vi "getSubM.vi"(9 "Index of Raws":T1, 11 "3D Array":dbl[][][](array[numeric])) -> (3 "Sub-Array":dbl[][][](array[numeric]))   [LabVIEW 2016]
doc: "Get the sub-matrix from a 3D matrix."
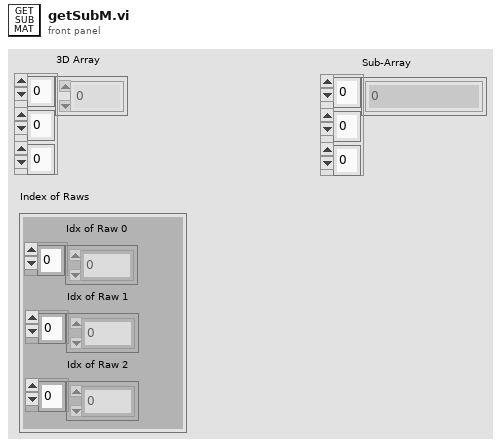
[diagram p1: front panel]
types:
  T1 = cluster{"Idx of Raw 0":i32[], "Idx of Raw 1":i32[], "Idx of Raw 2":i32[]}
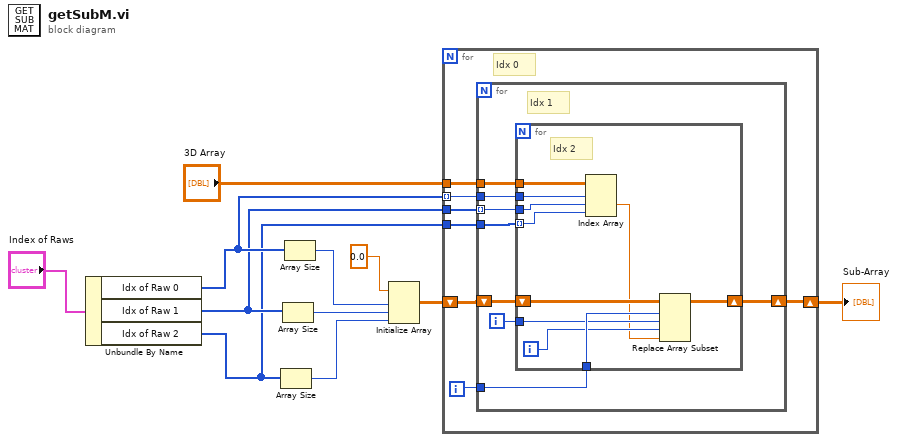
[diagram p0: block diagram]
diagram:
  n1 = Unbundle By Name("Index of Raws") -> ("Idx of Raw 0"=w3:i32[], "Idx of Raw 1"=w2:i32[], "Idx of Raw 2"=w1:i32[])
  n2 = Array Size(array=w1) -> (size(s)=w9:i32)
  n3 = Array Size(array=w2) -> (size(s)=w6:i32)
  n4 = Array Size(array=w3) -> (size(s)=w7:i32)
  n5 = Initialize Array(0.0 ("element"), w7, w6, w9) -> (w10:dbl[][][])
  n6 = for {
    tunnel: "3D Array" -> [w18]
    shift-right: [w16] -> w8
    shift-left: w10 -> [w17]
    tunnel: w3 -> [w15] mode=indexing
    tunnel: w2 -> [w14]
    tunnel: w1 -> [w13]
    i -> [w12]
    # "Idx 0"
    n7 = for {
      tunnel: w18 -> [w26]
      shift-right: [w24] -> w16
      shift-left: w17 -> [w25]
      tunnel: w15 -> [w23]
      tunnel: w14 -> [w22] mode=indexing
      tunnel: w13 -> [w21]
      tunnel: w12 -> [w20]
      i -> [w19]
      # "Idx 1"
      n8 = for {
        tunnel: w26 -> [w36]
        shift-right: [w30] -> w24
        shift-left: w25 -> [w32]
        tunnel: w23 -> [w35]
        tunnel: w22 -> [w34]
        tunnel: w21 -> [w33] mode=indexing
        tunnel: w20 -> [w31]
        tunnel: w19 -> [w29]
        i -> [w28]
        # "Idx 2"
        n9 = Index Array(array=w36, index (dim 0)=w35, index (dim 1)=w34, index (dim 2)=w33) -> (element=w27:dbl)
        n10 = Replace Array Subset(array=w32, new element=w27, index (dim 0)=w31, index (dim 1)=w29, index (dim 2)=w28) -> (w30:dbl[][][])
      }
    }
  }
  "Sub-Array" <- w8
